vi "sitios.vi"() -> ()   [LabVIEW 2010]
uses:
  <vilib>/addons/PixeLINK/Low Level Functions/CAMERA_FEATURES.llb/TDPU-CameraFeatures-PixelFormat.ctl
  <vilib>/Utility/error.llb/DialogType.ctl
  <vilib>/Utility/file.llb/Write To Spreadsheet File (DBL).vi
  <vilib>/vision/NI_Vision_Development_Module.lvlib
panel:
  out "Array":T1[](array[plugin-control])
  in  "Start":bool
  out "Image OUT":T1(plugin-control)
  out "new file path":path
  in  "nombre archivo":string
  in  "base path":path
  in  "Veces":i32
  in  "stop":bool
  in  "Valor Inicial":dbl
  in  "Tamaño del paso":dbl
  out "Imagenes tomadas":i32
  in  "tiempo entre pasos (ms)":dbl
  in  "Camara Parameters":T3 {"Pixel Format" items=["PIXEL_FORMAT_MONO8", "PIXEL_FORMAT_MONO16", "PIXEL_FORMAT_YUV422", "PIXEL_FORMAT_BAYER8_GRBG", "PIXEL_FORMAT_BAYER16_GRBG", "PIXEL_FORMAT_RGB24", "PIXEL_FORMAT_RGB48", "PIXEL_FORMAT_BAYER8_RGGB", "PIXEL_FORMAT_BAYER8_GBRG ", "PIXEL_FORMAT_BAYER8_BGGR ", "PIXEL_FORMAT_BAYER16_RGGB ", "PIXEL_FORMAT_BAYER16_GBRG", "PIXEL_FORMAT_BAYER16_BGGR", "PIXEL_FORMAT_RGB32"]}
  in  "Selector":u16(ring) items=["776002034"]
  in  "Streeam?":bool
  in  "DAQ Controls":T4={"Minimum Value"=-10.0, "Maximum Value"=10.0, "Physical Channel"="Dev1/ao0", "DAQ Fs (S/s)"=10000.0} {"Minimum Value" min=-10.0 max=0.0; "Maximum Value" min=0.0 max=10.0}
  in  "Imagenes":i32
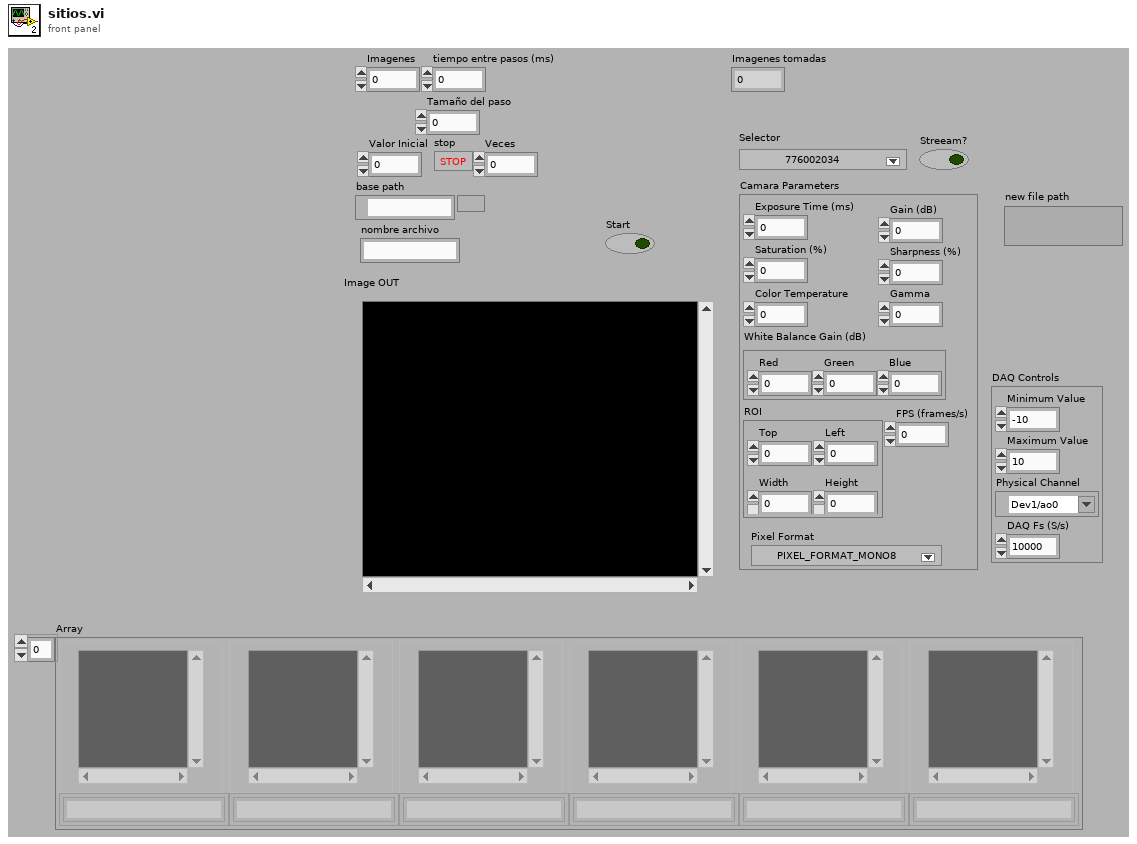
[diagram p1: front panel]
types:
  T1 = typedef "IMAQ Image.ctl" = refnum<image>
  T2 = typedef "TDPU-CameraFeatures-PixelFormat.ctl" = u16
  T3 = cluster{"Exposure Time (ms)":dbl, "Gain (dB)":dbl, "Saturation (%)":dbl, "Sharpness (%)":dbl, "Color Temperature":dbl, "ROI":cluster{"Top":i32, "Left":i32, "Width":i32, "Height":i32}, "White Balance Gain (dB)":cluster{"Red":dbl, "Green":dbl, "Blue":dbl}, "Gamma":dbl, "Pixel Format":T2, "FPS (frames/s)":i32}
  T4 = cluster{"Minimum Value":dbl, "Maximum Value":dbl, "Physical Channel":tag, "DAQ Fs (S/s)":dbl}
  T5 = cluster{"DAQ Fs (S/s)":dbl, "task":refnum<k21>, "error":errorcluster, "Min Value":dbl, "Max Value":dbl}
  T6 = cluster{"hCamera":u32, "Error":errorcluster, "uSerialNumber OUT":u32}
  T7 = cluster{"hCamera":u32, "Error":errorcluster, "uSerialNumber":u32}
  T8 = cluster{"DAQ Limits":cluster{"max":dbl, "min":dbl}, "Control Limits":cluster{"max":dbl, "min":dbl}}
  T9 = typedef "Image Type" = u32
  T10 = typedef "DialogType.ctl" = u16
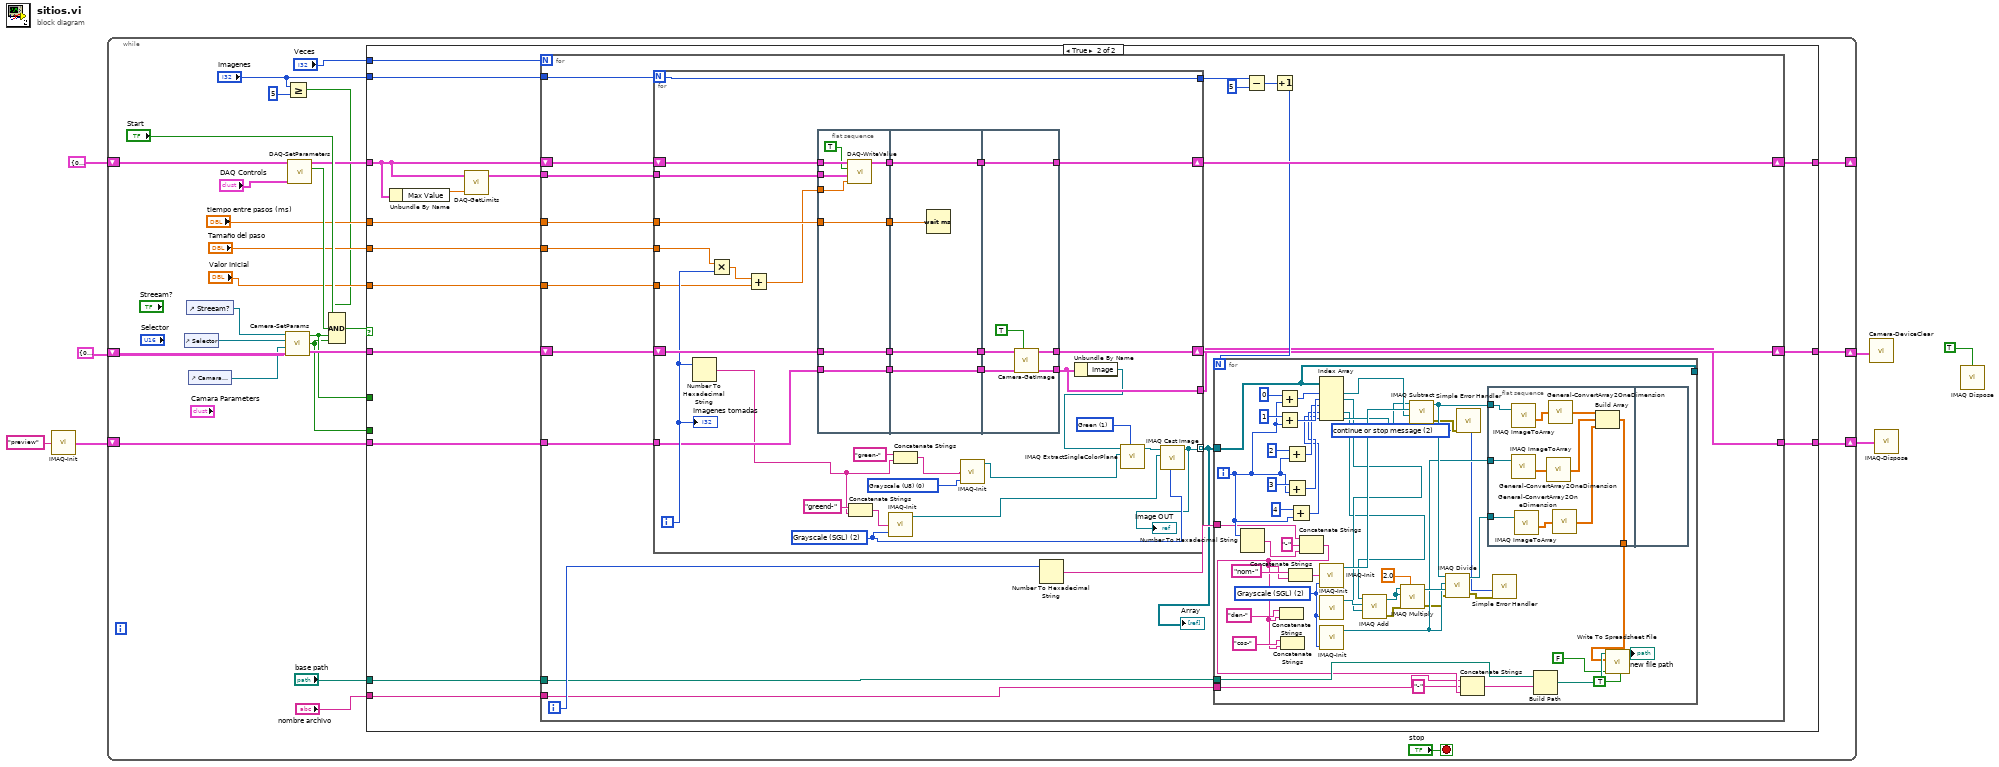
[diagram p0: block diagram]
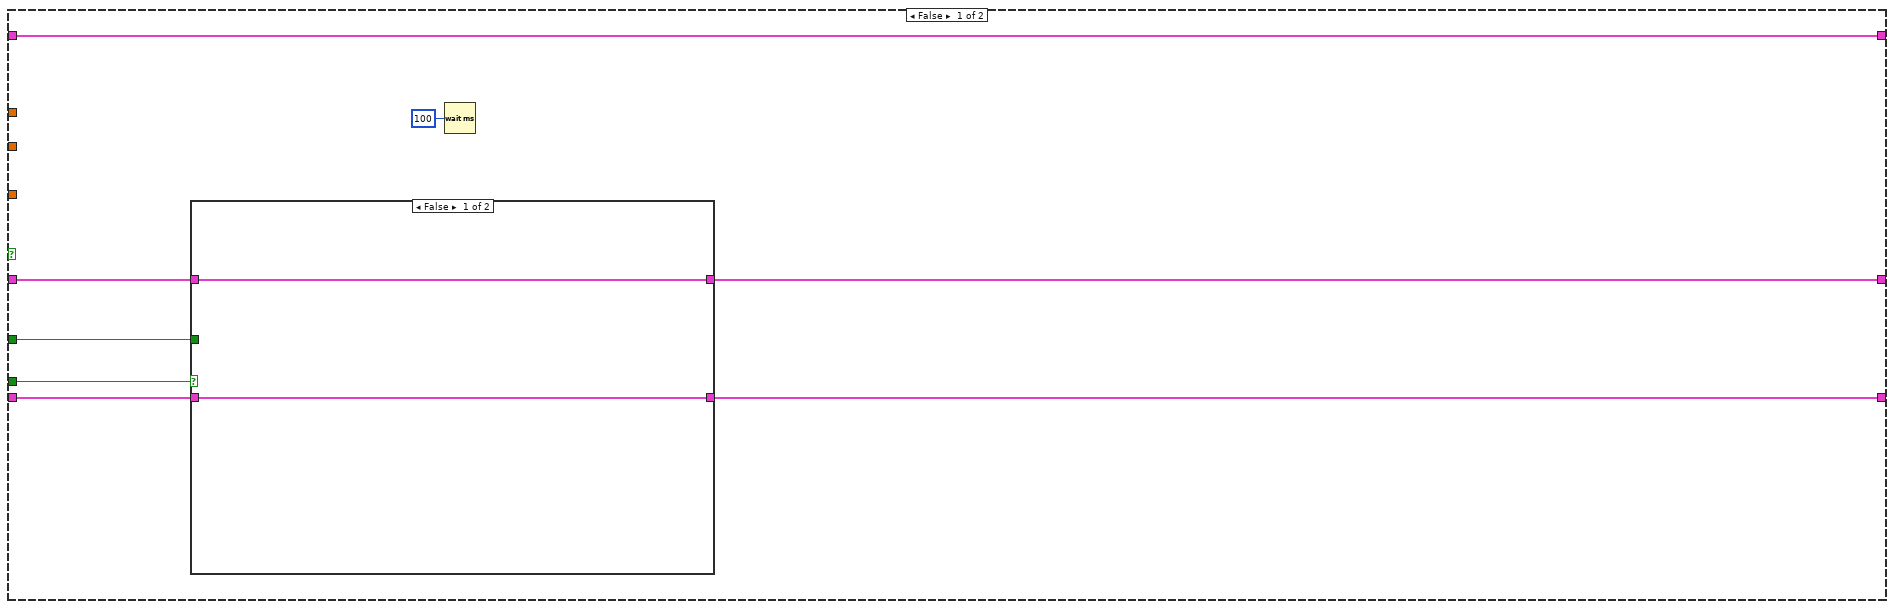
[diagram p2: hidden frame]
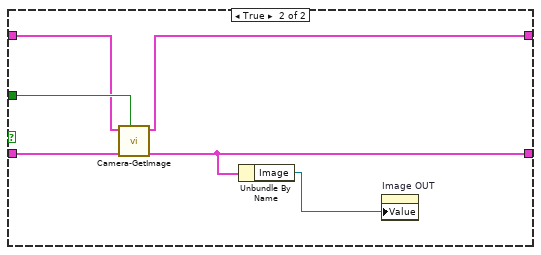
[diagram p3: hidden frame]
diagram:
  n1 = call "IMAQ-Init.vi"("Image Name"="preview") -> ("Image Device OUT"=w3:cluster{"Image":T1, "errorImage":errorcluster})  [unwired: 2 in, 2 out]
  n2 = while {
    shift-right: [w22] -> w1
    shift-left: T6 {"hCamera"=0, "Error"={"status"=FALSE, "code"=0, "source"=""}, "uSerialNumber OUT"=0} ("Camera Device  IN") -> [w29]
    shift-right: [w23] -> _
    shift-left: T5 {"DAQ Fs (S/s)"=0.0, "task"="", "error"={"status"=FALSE, "code"=0, "source"=""}, "Min Value"=0.0, "Max Value"=0.0} ("DAQ Device OUT") -> [w24]
    shift-right: [w9] -> w2
    shift-left: w3 -> [w11]
    stop <- "stop" stop-if-true
    n3 = control-ref of="Selector"() -> (w33:refnum<vi>)
    n4 = control-ref of="Streeam?"() -> (w32:refnum<vi>)
    n5 = control-ref of="Camara Parameters"() -> (w31:refnum<vi>)
    n6 = call "Camera-SetParams.vi"("Camera Device  IN"=w29, "Camera Parameters"=w31, "Selector"=w33, "Stream?"=w32) -> ("Camera Device OUT"=w30:T7, "Funciona?"=w8:bool, "Stream? OUT"=w10:bool)
    n7 = Greater Or Equal?(x="Imagenes", y=5) -> (x >= y?=w16:bool)
    n8 = call "DAQ-SetParameters.vi"("DAQ Controls"="DAQ Controls", "DAQ Device IN"=w24) -> ("En Funcionamiento?"=w27:bool, "DAQ Device OUT"=w25:T5)  [unwired: 4 in]
    n9 = Compound Arithmetic op=AND(w16, "Start", w27, w10, w8) -> (w28:bool)
    n10 = case shown="True" w28 {
      tunnel: w30 -> [w38 w65]
      tunnel: [w37 w56] -> w22
      tunnel: w25 -> [w41 w57]
      tunnel: [w41 w64] -> w23
      tunnel: "tiempo entre pasos (ms)" -> [_ w60]
      tunnel: "Imagenes" -> [_ w63]
      tunnel: "Tamaño del paso" -> [_ w59]
      tunnel: "Valor Inicial" -> [_ w58]
      tunnel: "Veces" -> [_ w55]
      tunnel: "base path" -> [_ w54]
      tunnel: "nombre archivo" -> [_ w53]
      tunnel: w11 -> [w40 w52]
      tunnel: w10 -> [w39 _]
      tunnel: [w36 w51] -> w9
      tunnel: w8 -> [w35 _]
      frame False {
        n11 = case shown="False" w35 {
          tunnel: w40 -> [w43 w50]
          tunnel: w39 -> [_ w49]
          tunnel: w38 -> [w44 w48]
          tunnel: [w44 w47] -> w37
          tunnel: [w43 w46] -> w36
          frame False {
          }
          frame True {
            n12 = call "Camera-GetImage.vi"("Streeam"=w49, "Image Device IN"=w50, "Camera Device IN"=w48) -> ("Image Device OUT"=w46:cluster{"Image":T1, "errorImage":errorcluster}, "Camera Device OUT"=w47:T7)  [unwired: 4 in]
            n13 = Unbundle By Name(w46) -> ("Image"=w45:T1)
            n14 = property on="Image OUT" class="ImageControl"("Value"=w45) -> ()  [unwired: 2 in, 2 out]
          }
        }
        n15 = Wait (ms)(milliseconds to wait=u32 100) -> ()  [unwired: 1 out]
      }
      frame True {
        n16 = Unbundle By Name(w57) -> ("Max Value"=w62:dbl)
        n17 = call "DAQ-GetLimits.vi"("Amplitud"=w62, "DAQ Device IN"=w57) -> ("Limites"=w61:T8)  [unwired: 3 in]
        n18 = for {
          N: w55 -> [_]
          tunnel: w63 -> [w83]
          tunnel: w61 -> [w82]
          tunnel: w60 -> [w81]
          tunnel: w59 -> [w80]
          tunnel: w58 -> [w79]
          shift-right: [w84] -> w64
          shift-left: w57 -> [w73]
          shift-right: [w72] -> w56
          shift-left: w65 -> [w85]
          tunnel: w54 -> [w70]
          tunnel: w53 -> [w69]
          tunnel: w52 -> [w68]
          tunnel: [w67] -> w51
          i -> [w71]
          n19 = for {
            N: w83 -> [w157]
            tunnel: w82 -> [w176]
            tunnel: w81 -> [w164]
            tunnel: w80 -> [w162]
            tunnel: w79 -> [w160]
            tunnel: [w143] -> w66 mode=indexing
            tunnel: [w157] -> w78
            shift-right: [w174] -> w84
            shift-left: w73 -> [w175]
            shift-right: [w168] -> w72
            shift-left: w85 -> [w171]
            tunnel: w68 -> [w154]
            tunnel: [w153] -> w67
            i -> [w163]
            w148 = T9 2 items=["Grayscale (U8)", "Grayscale (I16)", "Grayscale (SGL)", "Complex (CSG)", "RGB (U32)", "HSL (U32)", "RGB (U64)", "Grayscale (U16)"] ("Image Type")
            w152 = 1 items=["Red", "Green", "Blue", "Hue", "Saturation", "Luminance", "Value", "Intensity"] ("Color Plane")
            w155 = T9 0 items=["Grayscale (U8)", "Grayscale (I16)", "Grayscale (SGL)", "Complex (CSG)", "RGB (U32)", "HSL (U32)", "RGB (U64)", "Grayscale (U16)"] ("Image Type")
            n20 = Number To Hexadecimal String(2:w163) -> (0:w146:string)  [unwired: 1 in]
            n21 = Multiply(x=w162, y=w163) -> (x*y=w159:dbl)
            n22 = Add(x=w159, y=w160) -> (x+y=w161:dbl)
            n23 = flat-sequence {
              tunnel: w176 -> [w184]
              tunnel: w175 -> [w183]
              tunnel: [w182] -> w173
              tunnel: w171 -> [w181]
              tunnel: [w181] -> w169
              tunnel: [w180] -> w166
              tunnel: w154 -> [w180]
              tunnel: [w179] -> w165
              tunnel: w164 -> [w179]
              tunnel: w161 -> [w177]
              tunnel: w173 -> [w188]
              tunnel: [w188] -> w172
              tunnel: [w187] -> w170
              tunnel: w169 -> [w187]
              tunnel: [w186] -> w167
              tunnel: w166 -> [w186]
              tunnel: w165 -> [w185]
              tunnel: [w194] -> w174
              tunnel: w172 -> [w194]
              tunnel: w170 -> [w193]
              tunnel: [w192] -> w168
              tunnel: w167 -> [w191]
              tunnel: [w190] -> w153
              frame #0 {
                n24 = call "DAQ-WriteValue.vi"("Input"=w177, "Limites"=w184, "DAQ?"=TRUE, "DAQ Device IN"=w183) -> ("DAQ Device OUT"=w182:T5)  [unwired: 5 in]
              }
              frame #1 {
                n25 = Wait (ms)(milliseconds to wait=w185) -> ()  [unwired: 1 out]
              }
              frame #2 {
                n26 = call "Camera-GetImage.vi"("Streeam"=TRUE, "Image Device IN"=w191, "Camera Device IN"=w193) -> ("Image Device OUT"=w190:cluster{"Image":T1, "errorImage":errorcluster}, "Camera Device OUT"=w192:T7)  [unwired: 4 in]
              }
            }
            n27 = Concatenate Strings("greend-" ("string"), w146) -> (w145:string)
            n28 = call "IMAQ-Init.vi"("Image Type"=w148, "Image Name"=w145) -> ("Image OUT"=w149:T1)  [unwired: 1 in, 2 out]
            n29 = Concatenate Strings("green-" ("string"), w146) -> (w156:string)
            n30 = call "IMAQ-Init.vi"("Image Type"=w155, "Image Name"=w156) -> ("Image OUT"=w151:T1)  [unwired: 1 in, 2 out]
            n31 = Unbundle By Name(w153) -> ("Image"=w144:T1)
            n32 = call "IMAQ ExtractSingleColorPlane"("Color Plane"=w152, "Image Dst"=w151, "Image Src"=w144) -> ("Image Dst Out"=w150:T1)  [unwired: 7 in, 1 out]
            n33 = call "IMAQ Cast Image"("Image Type"=w148, "Image Dst"=w149, "Image Src"=w150) -> ("Image Dst Out"=w143:T1)  [unwired: 7 in, 1 out]
            "Image OUT" <- w143
            "Imagenes tomadas" <- w163
          }
          "Array" <- w66
          n34 = Number To Hexadecimal String(2:w71) -> (0:w74:string)  [unwired: 1 in]
          n35 = Subtract(x=w78, y=5) -> (x-y=w76:i32)
          n36 = Increment(x=w76) -> (x+1=w75:i32)
          n37 = for {
            N: w75 -> [_]
            tunnel: w66 -> [w114]
            tunnel: [w114] -> _
            tunnel: w74 -> [w110]
            tunnel: w70 -> [w105]
            tunnel: w69 -> [w96]
            i -> [w113]
            w86 = T10 2 items=["no dialog", "OK message", "continue or stop message", "OK message + warnings", "continue/stop + warnings"] ("type of dialog (OK msg:1)")
            w95 = T9 2 items=["Grayscale (U8)", "Grayscale (I16)", "Grayscale (SGL)", "Complex (CSG)", "RGB (U32)", "HSL (U32)", "RGB (U64)", "Grayscale (U16)"] ("Image Type")
            n38 = Number To Hexadecimal String(2:w113) -> (0:w111:string)  [unwired: 1 in]
            n39 = Add(x=0, y=w113) -> (x+y=w123:i32)
            n40 = Add(x=1, y=w113) -> (x+y=w122:i32)
            n41 = Add(x=2, y=w113) -> (x+y=w121:i32)
            n42 = Add(x=3, y=w113) -> (x+y=w120:i32)
            n43 = Add(x=4, y=w113) -> (x+y=w119:i32)
            n44 = Concatenate Strings(w110, "-" ("string"), w111) -> (w103:string)
            n45 = Concatenate Strings("den-" ("Image Name"), w103) -> ()  [unwired: 1 out]
            n46 = Concatenate Strings("cos-" ("Image Name"), w103) -> ()  [unwired: 1 out]
            n47 = Concatenate Strings("nom-" ("Image Name"), w103) -> (w127:string)
            n48 = Index Array(array=w114, index #1=w123, index #2=w122, index #3=w121, index #4=w120, index #5=w119) -> (element #1=w94:T1, element #2=w92:T1, element #4=w91:T1, element #5=w93:T1)  [unwired: 1 out]
            n49 = call "IMAQ-Init.vi"("Image Type"=w95, "Image Name"=w127) -> ("Image OUT"=w115:T1)  [unwired: 1 in, 2 out]
            n50 = call "IMAQ-Init.vi"("Image Type"=w95) -> ("Image OUT"=w117:T1)  [unwired: 2 in, 2 out]
            n51 = call "IMAQ-Init.vi"("Image Type"=w95) -> ("Image OUT"=w107:T1)  [unwired: 2 in, 2 out]
            n52 = call "IMAQ Add"("Image Src A"=w91, "Image Dst"=w117, "Image Src B"=w92) -> ("Image Dst Out"=w116:T1, "error out"=w90:errorcluster)  [unwired: 4 in]
            n53 = call "IMAQ Multiply"("Image Src A"=w116, "Constant"=sgl 2.0, "Image Dst"=w116, "error in (no error)"=w90) -> ("Image Dst Out"=w109:T1, "error out"=w89:errorcluster)  [unwired: 3 in]
            n54 = call "IMAQ Subtract"("Image Src A"=w93, "Image Dst"=w115, "Image Src B"=w94) -> ("Image Dst Out"=w108:T1, "error out"=w87:errorcluster)  [unwired: 4 in]
            n55 = call "IMAQ Divide"("Image Src A"=w108, "Image Dst"=w107, "Image Src B"=w109, "error in (no error)"=w89) -> ("Image Dst Out"=w106:T1, "error out"=w88:errorcluster)  [unwired: 3 in]
            n56 = call <vilib>:"Simple Error Handler.vi"("type of dialog (OK msg:1)"=w86, "error in (no error)"=w87) -> ()  [unwired: 3 in, 5 out]
            n57 = Concatenate Strings(w96, "-" ("string"), w103) -> (w104:string)
            n58 = flat-sequence {
              tunnel: w108 -> [w133]
              tunnel: w107 -> [w134]
              tunnel: w106 -> [w135]
              tunnel: [w136] -> w101
              frame #0 {
                n59 = call "IMAQ ImageToArray"("Image"=w134) -> ("Image Pixels (Float)"=w140:sgl[][])  [unwired: 3 in, 4 out]
                n60 = call "IMAQ ImageToArray"("Image"=w133) -> ("Image Pixels (Float)"=w142:sgl[][])  [unwired: 3 in, 4 out]
                n61 = call "IMAQ ImageToArray"("Image"=w135) -> ("Image Pixels (Float)"=w139:sgl[][])  [unwired: 3 in, 4 out]
                n62 = call "General-ConvertArray2OneDimension.vi"("Input Array"=w140) -> ("Output Array"=w138:dbl[])
                n63 = call "General-ConvertArray2OneDimension.vi"("Input Array"=w142) -> ("Output Array"=w141:dbl[])
                n64 = call "General-ConvertArray2OneDimension.vi"("Input Array"=w139) -> ("Output Array"=w137:dbl[])
                n65 = Build Array(w141, w138, w137) -> (w136:dbl[][])
              }
              frame #1 {
              }
            }
            n66 = call <vilib>:"Simple Error Handler.vi"("type of dialog (OK msg:1)"=w86, "error in (no error)"=w88) -> ()  [unwired: 3 in, 5 out]
            n67 = Build Path(base path=w105, name or relative path=w104) -> (appended path=w102:path)
            n68 = call-poly <vilib>:"Write To Spreadsheet File.vi"("transpose? (no:F)"=TRUE, "append to file? (new file:F)"=FALSE, "2D data"=w101, "file path (dialog if empty)"=w102) -> ("new file path (Not A Path if cancelled)"=→"new file path":path)  [unwired: 4 in]
          }
        }
      }
    }
  }
  n69 = call "Camera-DeviceClear.vi"("Camera Device OUT"=w1) -> ()
  n70 = call "IMAQ-Dispose.vi"("Image Device IN"=w2) -> ()
  n71 = call "IMAQ Dispose"("All Images? (No)"=TRUE) -> ()  [unwired: 5 in, 1 out]
